vi "TestVisibility.vi"(8 "error in":errorcluster) -> (0 "error out":errorcluster)   [LabVIEW 2016, in "WeatherReportTests.lvlib"]
uses:
  WeatherReportTests.lvlib
  APIs/Stimulus/ControlValue/SetValueAuto.vi
  APIs/Stimulus/ControlValue/Controls/Tree/SetValueByHierarchicalPath.vi
  APIs/Stimulus/ControlValue/Controls/Listbox/SetValueByItemName.vi
  APIs/Assert/AssertControlProperty/AssertControlVisible/AssertVisible.vi
  APIs/Assert/AssertControlProperty/AssertControlVisible/AssertInvisible.vi
  APIs/Stimulus/VI/CloseVI.vi
  Drona.lvlib
  <vilib>/addons/_JKI Toolkits/Caraya/classes/Test/Test.lvclass
  APIs/Stimulus/ControlValue/Controls/Listbox/StimulusListbox.lvlib
  APIs/Stimulus/ControlValue/ControlValue.lvlib
  APIs/Stimulus/ControlValue/Controls/Tree/StimulusTree.lvlib
  APIs/Stimulus/VI/VI.lvlib
  APIs/Assert/AssertControlProperty/AssertControlVisible/AssertControlVisible.lvlib
panel:
  # "Drona Test Visibility"
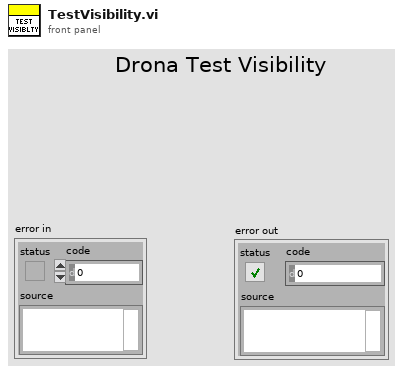
[diagram p1: front panel]
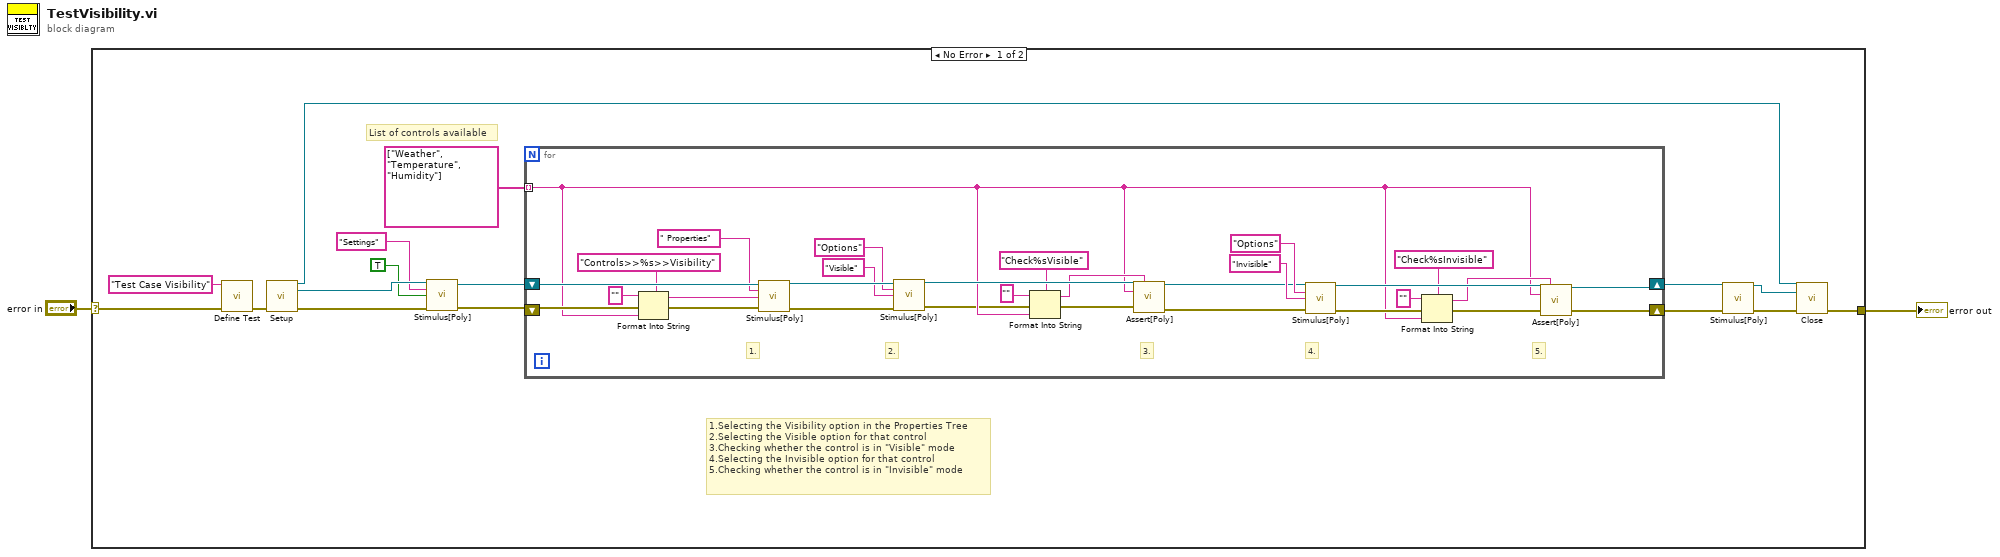
[diagram p0: block diagram]
diagram:
  n1 = case shown="No Error" "error in" {
    selector: "error in" -> [w16 w49]
    tunnel: [w5 w49] -> w1
    frame No Error {
      # "1.Selecting the Visibility option in the Properties Tree\n2.Selecting the Visible option for that control\n3.Checking whether the control is in \"Visible\" mode\n4.Selecting the Invisible option for that control\n5.Checking whether the control is in \"Invisible\" mode"
      # "List of controls available"
      n2 = call <vilib>:"Define Test.vi"("error in (no error)"=w16, "Label (VI Title)"="Test Case Visibility") -> ("error out"=w18:errorcluster)  [unwired: 8 in, 1 out]
      n3 = call "Setup.vi"("error in"=w18) -> ("Application Ref"=w6:refnum<vi>, "VI Reference Out"=w15:refnum<vi>, "error out"=w14:errorcluster)  [unwired: 12 in]
      n4 = call-poly "Stimulus[Poly].vi"("VI Reference In"=w15, "Control Path"="Settings", "Value (Signaling)"=TRUE, "error in"=w14) -> ("VI Reference Out"=w10:refnum<vi>, "error out"=w11:errorcluster)  [unwired: 10 in]
      n5 = for {
        tunnel: string[] ["Weather", "Temperature", "Humidity"] ("Control Path") -> [w24] mode=indexing
        shift-right: [w36] -> w4
        shift-left: w11 -> [w48]
        shift-right: [w19] -> w9
        shift-left: w10 -> [w47]
        # "5."
        # "4."
        # "3."
        # "2."
        # "1."
        n6 = Format Into String(format string="Controls>>%s>>Visibility" ("Control Path"), initial string="", error in=w48, w24) -> (resulting string=w33:string, error out=w35:errorcluster)
        n7 = call-poly "Stimulus[Poly].vi"("VI Reference In"=w47, "Control Path"=" Properties", "Hierarchical Path"=w33, "Error In"=w35) -> ("VI Reference Out"=w45:refnum<vi>, "Error Out"=w23:errorcluster)  [unwired: 10 in]
        n8 = call-poly "Stimulus[Poly].vi"("VI Reference In"=w45, "Control Path"="Options", "Item Name"="Visible", "Error In"=w23) -> ("VI Reference Out"=w42:refnum<vi>, "Error Out"=w22:errorcluster)  [unwired: 10 in]
        n9 = Format Into String(format string="Check%sVisible" ("Label"), initial string="", error in=w22, w24) -> (resulting string=w26:string, error out=w21:errorcluster)
        n10 = call-poly "Assert[Poly].vi"("VI Reference In"=w42, "Label"=w26, "Control Path"=w24, "Error In"=w21) -> ("VI Reference Out"=w20:refnum<vi>, "Error Out"=w37:errorcluster)  [unwired: 9 in, 1 out]
        n11 = call-poly "Stimulus[Poly].vi"("VI Reference In"=w20, "Control Path"="Options", "Item Name"="Invisible", "Error In"=w37) -> ("VI Reference Out"=w40:refnum<vi>, "Error Out"=w41:errorcluster)  [unwired: 10 in]
        n12 = Format Into String(format string="Check%sInvisible" ("Label"), initial string="", error in=w41, w24) -> (resulting string=w25:string, error out=w32:errorcluster)
        n13 = call-poly "Assert[Poly].vi"("VI Reference In"=w40, "Label"=w25, "Control Path"=w24, "Error In"=w32) -> ("VI Reference Out"=w19:refnum<vi>, "Error Out"=w36:errorcluster)  [unwired: 9 in, 1 out]
      }
      n14 = call-poly "Stimulus[Poly].vi"("VI Reference In"=w9, "error in"=w4) -> ("VI Reference Out"=w8:refnum<vi>, "error out"=w7:errorcluster)  [unwired: 12 in]
      n15 = call "Close.vi"("Application Ref"=w6, "VI Reference"=w8, "error in"=w7) -> ("error out"=w5:errorcluster)  [unwired: 12 in]
    }
    frame Error {
    }
  }
  "error out" <- w1
